vi "PH_BeamlineController.PC Set-Source.vi"(0 "i ref in":refnum<vi>, 2 "Source":T1, 3 "Value":bool, 5 "error in (no error)":errorcluster) -> (14 "i ref out":refnum<vi>, 17 "Sources changed?":bool, 19 "error out":errorcluster)   [LabVIEW 2014, in "PH_BeamlineController.lvlib"]
doc: "This VI writes incoming Information to own Attributes if the new value differs from the stored."
uses:
  PH_BeamlineController.lvlib
  PH_BeamlineController.Sources.ctl
  PH_Basics/PH_SystemInformation/PH_SystemInformationEnabling State.ctl
  PH_Basics/PH_SystemInformation/PH_SystemInformation.lvlib
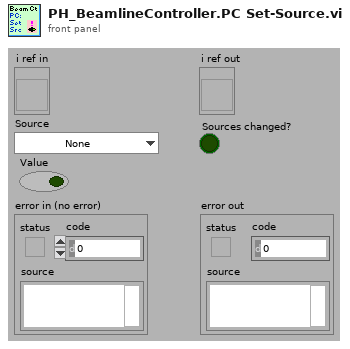
[diagram p1: front panel]
types:
  T1 = typedef "PH_BeamlineController.lvlib/PH_BeamlineController.Sources.ctl" = enum16{"None", "YLF", "fs-Frontend", "ns-Frontend", "YLF and ns-Frontend", "fs- and ns-Frontend"}
  T2 = typedef "PH_SystemInformation.lvlib/PH_SystemInformationEnabling State.ctl" = i32
  T3 = enum16{"Laser", "PreAmp", "MainAmp", "Exp 1", "Exp 2", "Exp 3", "Exp 4"}
  T4 = typedef "PH_BeamlineController.lvlib/PH_BeamlineController.Source Attributes.ctl" = cluster{"Name":T1, "GUI Ref":refnum<vi>, "Current State":bool, "Wanted State":bool}
  T5 = typedef "PH_BeamlineController.lvlib/PH_BeamlineController.PA DP Targets.ctl" = enum16{"None", "Dump PA Delayed Beam", "Dump PA Undelayed Beam", "Dumps PA Delayed and Undelayed Beam"}
  T6 = typedef "PH_BeamlineController.lvlib/PH_BeamlineController.i attribute.ctl" = cluster{"Vacuum Exp LB":cluster{"Channel":string, "Limit [mbar]":dbl, "Pressure [mbar]":dbl, "GUI Ref":refnum<vi>}, "Sources":T4[], "PA DP Targets":T7[], "Path":cluster{"Source":T1, "PA DP Target":T5, "Target":T8}, "Targets":cluster{"Name":T8, "GUI Ref":refnum<vi>, "Current State":bool, "Wanted State":bool, "Enabled":bool}[], "Status Tags":cluster{"Name":string, "Status":T9}[], "special GUI Refs":T10}
  T7 = typedef "PH_BeamlineController.lvlib/PH_BeamlineController.PA DP Target Attributes.ctl" = cluster{"Name":T5, "GUI Ref":refnum<vi>, "Current State":bool, "Wanted State":bool, "Enabled":bool}
  T8 = typedef "PH_BeamlineController.lvlib/PH_BeamlineController.Targets.ctl" = enum16{"None", "PreAmp", "Dump Exp Laserlab", "Exp Laserlab", "Calorimeter", "Dump Exp Laserbay", "Exp Laserbay", "Dump Exp Z6", "Exp Z6"}
  T9 = typedef "PH_StatusHandler.lvlib/PH_StatusHandler.Status.ctl" = i16
  T10 = typedef "PH_BeamlineController.lvlib/PH_BeamlineController.special GUI Refs.ctl" = cluster{"PA-Backreflection-Meas":refnum<vi>, "fs_Synchrolock_Watch":refnum<vi>}
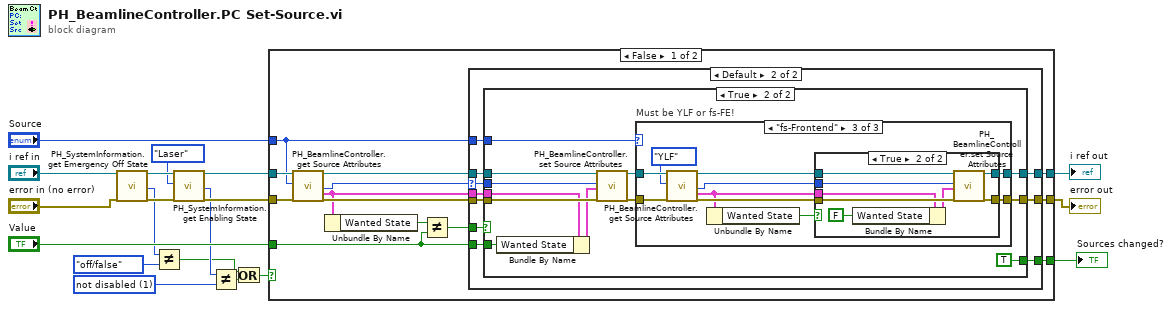
[diagram p0: block diagram]
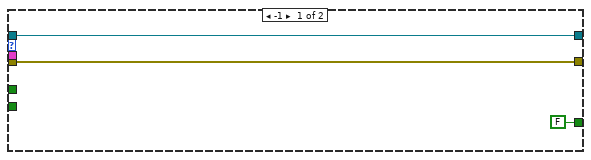
[diagram p2: hidden frame]
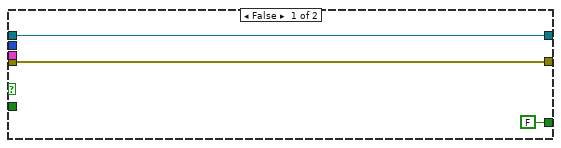
[diagram p3: hidden frame]
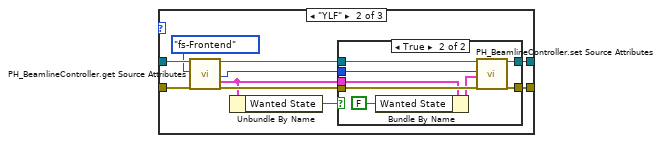
[diagram p5: hidden frame]
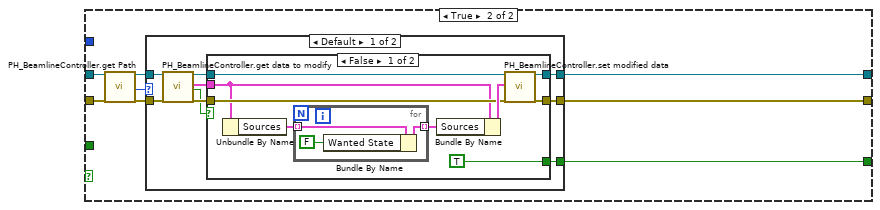
[diagram p8: hidden frame]
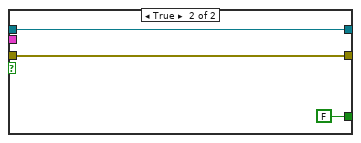
[diagram p9: hidden frame]
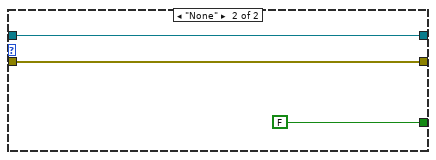
[diagram p10: hidden frame]
diagram:
  w4 = T2 1 items=["no info", "not disabled", "disabled"] ("y")
  n1 = call "PH_SystemInformation.get Emergency Off State.vi"("i ref in"="i ref in", "error in (no error)"="error in (no error)") -> ("i ref out"=w15:refnum<vi>, "Emergency Off State"=w7:enum16{"no info", "off/false", "Alarm"}, "error out"=w13:errorcluster)  [unwired: 15 in]
  n2 = Not Equal?(x=w7, y=enum16{"no info", "off/false", "Alarm"}."off/false") -> (x != y?=w3:bool)
  n3 = call "PH_SystemInformation.get Enabling State.vi"("i ref in"=w15, "Wanted State"=T3."Laser", "error in (no error)"=w13) -> ("i ref out"=w14:refnum<vi>, "Enabling State"=w5:T2, "error out"=w12:errorcluster)  [unwired: 14 in]
  n4 = Not Equal?(x=w5, y=w4) -> (x != y?=w2:bool)
  n5 = Or(x=w3, y=w2) -> (x .or. y?=w1:bool)
  n6 = case shown="False" w1 {
    tunnel: [w32 w105] -> w19
    tunnel: [w31 w106] -> w18
    tunnel: w14 -> [w28 w110]
    tunnel: w12 -> [w27 w109]
    tunnel: "Source" -> [w23 _]
    tunnel: [w22 w104] -> w9
    tunnel: "Value" -> [w20 _]
    frame False {
      n7 = call "PH_BeamlineController.get Source Attributes.vi"("VI in"=w28, "Source"=w23, "error in (no error)"=w27) -> ("VI out"=w29:refnum<vi>, "Source Index"=w21:i32, "Source Attributes"=w26:T4, "error out"=w30:errorcluster)  [unwired: 13 in]
      n8 = Unbundle By Name(w26) -> ("Wanted State"=w25:bool)
      n9 = Not Equal?(x=w25, y=w20) -> (x != y?=w24:bool)
      n10 = case shown="Default" w21 {
        selector: w21 -> [_ w36]
        tunnel: [w34 w45] -> w32
        tunnel: [w35 w44] -> w31
        tunnel: w30 -> [w34 w43]
        tunnel: w29 -> [w35 w42]
        tunnel: w20 -> [_ w41]
        tunnel: w26 -> [_ w40]
        tunnel: w24 -> [_ w39]
        tunnel: w23 -> [_ w38]
        tunnel: [FALSE w37] -> w22
        frame -1 {
        }
        frame Default {
          n11 = case shown="True" w39 {
            tunnel: [w48 w53] -> w44
            tunnel: [w47 w51] -> w45
            tunnel: w43 -> [w47 w60]
            tunnel: w42 -> [w48 w59]
            tunnel: w36 -> [_ w58]
            tunnel: w40 -> [_ w57]
            tunnel: w41 -> [_ w55]
            tunnel: w38 -> [_ w50]
            tunnel: [FALSE TRUE] -> w37
            frame False {
            }
            frame True {
              n12 = Bundle By Name(cluster=w57, "Wanted State"=w55) -> (w56:T4)
              n13 = call "PH_BeamlineController.set Source Attributes.vi"("VI in"=w59, "Source Index"=w58, "Changed Source Attributes"=w56, "error in (no error)"=w60) -> ("VI out"=w54:refnum<vi>, "error out"=w52:errorcluster)  [unwired: 14 in]
              n14 = case "Must be YLF or fs-FE!" shown="\"fs-Frontend\"" w50 {
                tunnel: w54 -> [w62 w71 w91]
                tunnel: [w62 w70 w90] -> w53
                tunnel: w52 -> [w61 w68 w88]
                tunnel: [w61 w67 w87] -> w51
                frame Default {
                }
                frame "YLF" {
                  n15 = call "PH_BeamlineController.get Source Attributes.vi"("VI in"=w71, "Source"=PH_BeamlineController.Sources."fs-Frontend", "error in (no error)"=w68) -> ("VI out"=w72:refnum<vi>, "Source Index"=w63:i32, "Source Attributes"=w64:T4, "error out"=w69:errorcluster)  [unwired: 13 in]
                  n16 = Unbundle By Name(w64) -> ("Wanted State"=w65:bool)
                  n17 = case shown="True" w65 {
                    tunnel: w72 -> [w74 w82]
                    tunnel: [w74 w81] -> w70
                    tunnel: w69 -> [w73 w80]
                    tunnel: [w73 w79] -> w67
                    tunnel: w64 -> [_ w78]
                    tunnel: w63 -> [_ w75]
                    frame False {
                    }
                    frame True {
                      n18 = Bundle By Name(cluster=w78, "Wanted State"=FALSE) -> (w77:T4)
                      n19 = call "PH_BeamlineController.set Source Attributes.vi"("VI in"=w82, "Source Index"=w75, "Changed Source Attributes"=w77, "error in (no error)"=w80) -> ("VI out"=w81:refnum<vi>, "error out"=w79:errorcluster)  [unwired: 14 in]
                    }
                  }
                }
                frame "fs-Frontend" {
                  n20 = call "PH_BeamlineController.get Source Attributes.vi"("VI in"=w91, "Source"=PH_BeamlineController.Sources."YLF", "error in (no error)"=w88) -> ("VI out"=w92:refnum<vi>, "Source Index"=w83:i32, "Source Attributes"=w84:T4, "error out"=w89:errorcluster)  [unwired: 13 in]
                  n21 = Unbundle By Name(w84) -> ("Wanted State"=w85:bool)
                  n22 = case shown="True" w85 {
                    tunnel: w92 -> [w94 w102]
                    tunnel: [w94 w101] -> w90
                    tunnel: w89 -> [w93 w100]
                    tunnel: [w93 w99] -> w87
                    tunnel: w84 -> [_ w98]
                    tunnel: w83 -> [_ w95]
                    frame False {
                    }
                    frame True {
                      n23 = Bundle By Name(cluster=w98, "Wanted State"=FALSE) -> (w97:T4)
                      n24 = call "PH_BeamlineController.set Source Attributes.vi"("VI in"=w102, "Source Index"=w95, "Changed Source Attributes"=w97, "error in (no error)"=w100) -> ("VI out"=w101:refnum<vi>, "error out"=w99:errorcluster)  [unwired: 14 in]
                    }
                  }
                }
              }
            }
          }
        }
      }
    }
    frame True {
      n25 = call "PH_BeamlineController.get Path.vi"("VI in"=w110, "error in (no error)"=w109) -> ("VI out"=w108:refnum<vi>, "Path:  PA DP Targets"=w103:T5, "error out"=w107:errorcluster)  [unwired: 12 in, 3 out]
      n26 = case shown="Default" w103 {
        tunnel: w108 -> [w115 w137]
        tunnel: w107 -> [w113 w136]
        tunnel: [w114 w137] -> w106
        tunnel: [w112 w136] -> w105
        tunnel: [w111 FALSE] -> w104
        frame Default {
          n27 = call "PH_BeamlineController.get data to modify.vi"("i ref in"=w115, "error in (no error)"=w113) -> ("i ref out"=w119:refnum<vi>, "i attribute"=w117:T6, "timed out"=w116:bool, "error out"=w118:errorcluster)  [unwired: 14 in]
          n28 = case shown="False" w116 {
            tunnel: w119 -> [w125 w134]
            tunnel: [w128 w134] -> w114
            tunnel: w118 -> [w124 w133]
            tunnel: [w127 w133] -> w112
            tunnel: w117 -> [w123 _]
            tunnel: [TRUE FALSE] -> w111
            frame False {
              n29 = Unbundle By Name(w123) -> ("Sources"=w122:T4[])
              n30 = for {
                tunnel: w122 -> [w131] mode=indexing
                tunnel: [w130] -> w121 mode=indexing
                n31 = Bundle By Name(cluster=w131, "Wanted State"=FALSE) -> (w130:T4)
              }
              n32 = Bundle By Name(cluster=w123, "Sources"=w121) -> (w126:T6)
              n33 = call "PH_BeamlineController.set modified data.vi"("i ref in"=w125, "i attribute"=w126, "error in (no error)"=w124) -> ("i ref out"=w128:refnum<vi>, "error out"=w127:errorcluster)  [unwired: 15 in]
            }
            frame True {
            }
          }
        }
        frame "None" {
        }
      }
    }
  }
  "error out" <- w19
  "i ref out" <- w18
  "Sources changed?" <- w9
